vi "Main.vi"(8 "error in (no error)":errorcluster, 11 "FactoryMethodDemo":refnum<class "ClientDemo.lvclass">) -> (0 "error out":errorcluster, 3 "FactoryMethodDemo":refnum<class "ClientDemo.lvclass">)   [LabVIEW 2020, in "FactoryMethod.lvlib" / "NoParametrizedFactoryMethod.lvlib" / "ClientDemo.lvclass"]
uses:
  ClientDemo.lvclass
  EnchantedMazeGame/EnchantedMazeGame.lvclass
  E:/GitHub/Design-Patterns-GoF_-_NI-LV/Creational/FactoryMethod/GoF_Example/NoParametrizedFactoryMethod/MazeGame/MazeGame.lvclass
  GoFcommonClasses/Maze/Maze.lvclass
  MazeGame/MazeGame.lvclass
  Support/Class/ConsoleOutput.lvclass
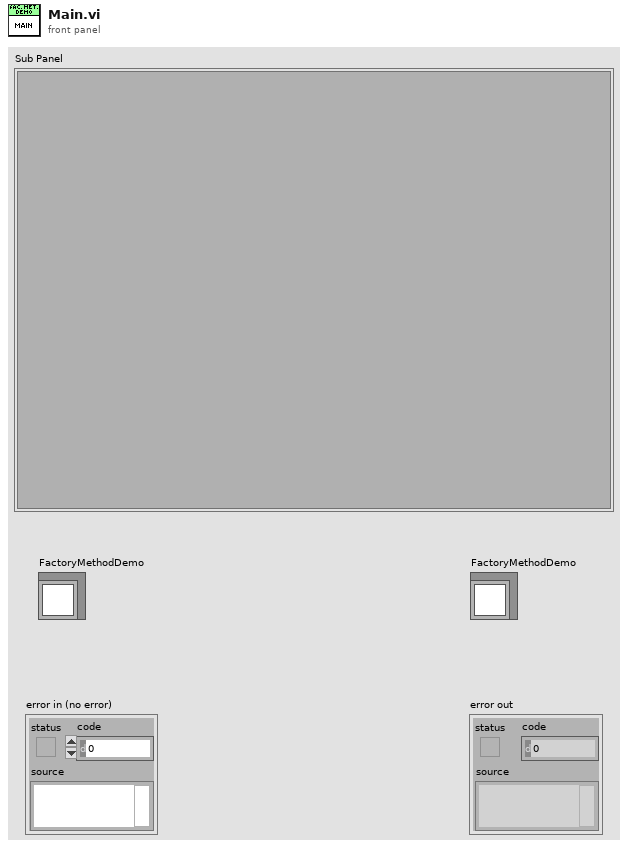
[diagram p1: front panel]
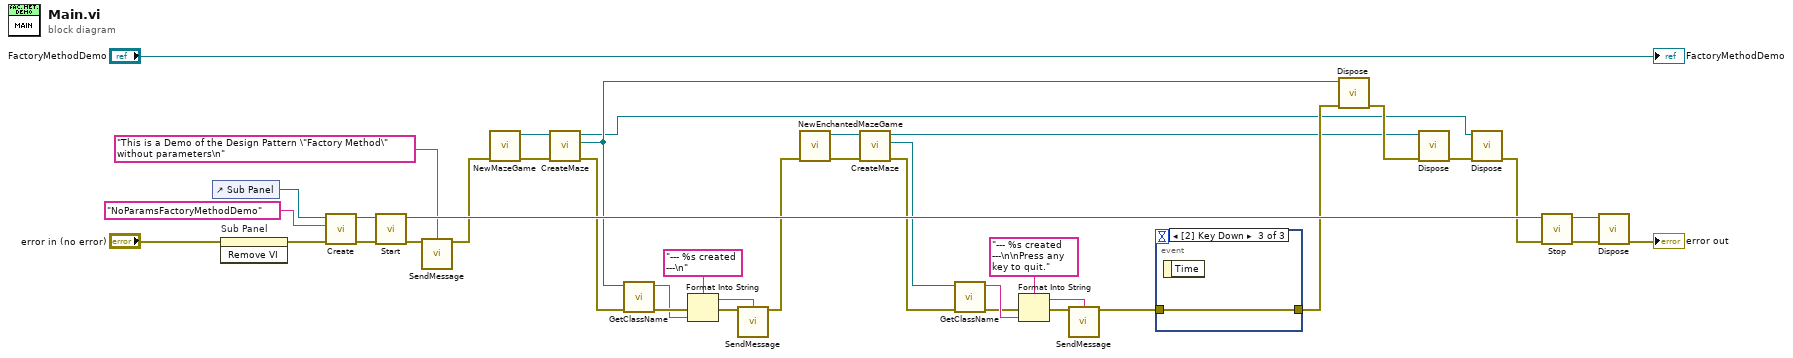
[diagram p0: block diagram]
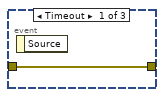
[diagram p2: hidden frame]
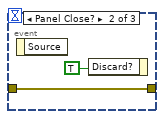
[diagram p3: hidden frame]
diagram:
  n1 = control-ref of="Sub Panel"() -> (w32:refnum<vi>)
  n2 = invoke on="Sub Panel" class="SubPnl" method="Remove VI"(error in="error in (no error)") -> (error out=w33:errorcluster)  [unwired: 2 in, 2 out]
  n3 = call "Create.vi"("error in (no error)"=w33, "LoggerName"="NoParamsFactoryMethodDemo", "SubPanelRef"=w32) -> ("error out"=w40:errorcluster, "ConsoleOutput out"=w39:refnum<class "ConsoleOutput.lvclass">)  [unwired: 7 in]
  n4 = call "Start.vi"("error in (no error)"=w40, "ConsoleOutput in"=w39) -> ("error out"=w34:errorcluster, "ConsoleOutput out"=w36:refnum<class "ConsoleOutput.lvclass">)  [unwired: 8 in]
  n5 = call "SendMessage.vi"("Message"="This is a Demo of the Design Pattern \"Factory Method\" without parameters\n" ("Data"), "error in (no error)"=w34) -> ("error out"=w29:errorcluster)  [unwired: 13 in]
  n6 = call "NewMazeGame.vi"("error in (no error)"=w29) -> ("error out"=w28:errorcluster, "MazeGame"=w27:refnum<class "MazeGame.lvclass">)  [unwired: 9 in]
  n7 = call "CreateMaze.vi"("error in (no error)"=w28, "MazeGame in"=w27) -> ("error out"=w16:errorcluster, "Maze"=w18:refnum<class "Maze.lvclass">, "MazeGame out"=w1:refnum<class "MazeGame.lvclass">)  [unwired: 7 in]
  n8 = call "GetClassName.vi"("error in (no error)"=w16, "object"=w18) -> ("error out"=w26:errorcluster, "Class Name"=w25:string)  [unwired: 8 in]
  n9 = Format Into String(format string="--- %s created ---\n", error in=w26, w25) -> (resulting string=w22:string, error out=w23:errorcluster)  [unwired: 1 in]
  n10 = call "SendMessage.vi"("Message"=w22, "error in (no error)"=w23) -> ("error out"=w13:errorcluster)  [unwired: 13 in]
  n11 = call "NewEnchantedMazeGame.vi"("error in (no error)"=w13) -> ("error out"=w15:errorcluster, "MazeGame"=w14:refnum<class "EnchantedMazeGame.lvclass">)  [unwired: 9 in]
  n12 = call "CreateMaze.vi"("error in (no error)"=w15, "MazeGame in"=w14) -> ("error out"=w7:errorcluster, "Maze"=w6:refnum<class "Maze.lvclass">, "MazeGame out"=w2:refnum<class "EnchantedMazeGame.lvclass">)  [unwired: 7 in]
  n13 = call "GetClassName.vi"("error in (no error)"=w7, "object"=w6) -> ("error out"=w8:errorcluster, "Class Name"=w9:string)  [unwired: 8 in]
  n14 = Format Into String(format string="--- %s created ---\n\nPress any key to quit.", error in=w8, w9) -> (resulting string=w12:string, error out=w11:errorcluster)  [unwired: 1 in]
  n15 = call "SendMessage.vi"("Message"=w12, "error in (no error)"=w11) -> ("error out"=w5:errorcluster)  [unwired: 13 in]
  n16 = event shown="[2] Key Down" {
    selector: _ -> [_ _ _]
    dyn-events: _ -> [_ _ _]
    timeout: _ -> [_ _ _]
    tunnel: w5 -> [w41 w43 w44]
    tunnel: [w41 w43 w44] -> w17
    event Timeout {
      n17 = event-data() -> ()  [unwired: 1 in, 1 out]
    }
    event Panel Close? {
      n18 = event-data() -> ()  [unwired: 1 in, 1 out]
      n19 = event-data("Discard?"=TRUE) -> ()  [unwired: 1 in, 1 out]
    }
    event Key Down {
      n20 = event-data() -> ()  [unwired: 1 in, 1 out]
    }
  }
  n21 = call-dynamic "Dispose.vi"("error in (no error)"=w17, "Maze"=w18) -> ("error out"=w3:errorcluster)  [unwired: 9 in]
  n22 = call-dynamic "Dispose.vi"("error in (no error)"=w3, "ByRef"=w2) -> ("error out"=w4:errorcluster)  [unwired: 9 in]
  n23 = call-dynamic "Dispose.vi"("error in (no error)"=w4, "ByRef"=w1) -> ("error out"=w19:errorcluster)  [unwired: 9 in]
  n24 = call "Stop.vi"("error in (no error)"=w19, "ConsoleOutput in"=w36) -> ("error out"=w21:errorcluster, "ConsoleOutput out"=w37:refnum<class "ConsoleOutput.lvclass">)  [unwired: 8 in]
  n25 = call "Dispose.vi"("error in (no error)"=w21, "ConsoleOutput in"=w37) -> ("error out"=→"error out":errorcluster)  [unwired: 9 in]
  "FactoryMethodDemo" <- "FactoryMethodDemo"
